vi "Single Ch PI Connect Sequence.vi"(8 "error in (no error)":errorcluster) -> (0 "error out":errorcluster, 2 "PreLaunchStagePos":T1={"Position (SET)"={"XaxesSET"=0.0}, "Position (ACT)"={"PosXACT"=0.0087}} caption="output cluster" {"Position (ACT)"."PosXACT" min=0.0 max=220.0 step=0.1 format="%.2f"; "Position (SET)"."XaxesSET" min=0.0 max=220.0 step=0.1 scale=0.0..220.0}, 3 "Boolean":bool)   [LabVIEW 2020]
uses:
  PI Settings.ctl
  PI Settings Global.vi
  Low Level/Communication.llb/Global1.vi
  Low Level/Communication.llb/Available DLL interfaces.ctl
  Low Level/Communication.llb/Available DLLs.ctl
  Single Ch PI Position.ctl
panel:
  out "Conn. Axes":string[](array[string])
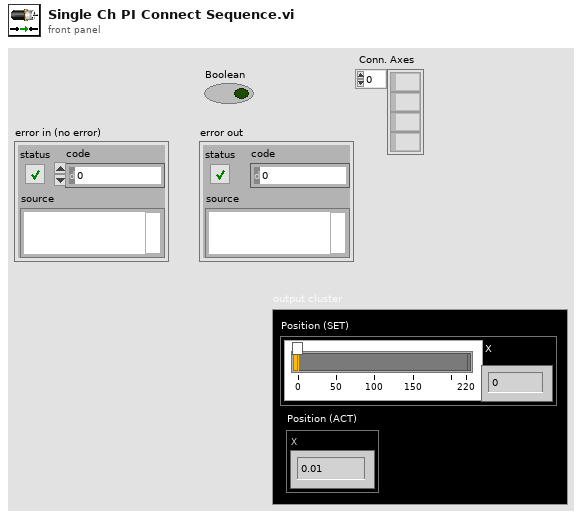
[diagram p1: front panel]
types:
  T1 = typedef "Single Ch PI Position.ctl" = cluster{"Position (SET)":cluster{"XaxesSET":dbl}, "Position (ACT)":cluster{"PosXACT":dbl}}
  T2 = typedef "PI Settings.ctl" = cluster{"System number":i32, "Commanded axes":string[], "Controller error":bool, "Error":errorcluster}
  T3 = typedef "Available DLLs.ctl" = u16
  T4 = typedef "Available DLL interfaces.ctl" = u16
  T5 = cluster{"DLL for Device":T3, "DLL Interface":T4, "Parameter":string}[]
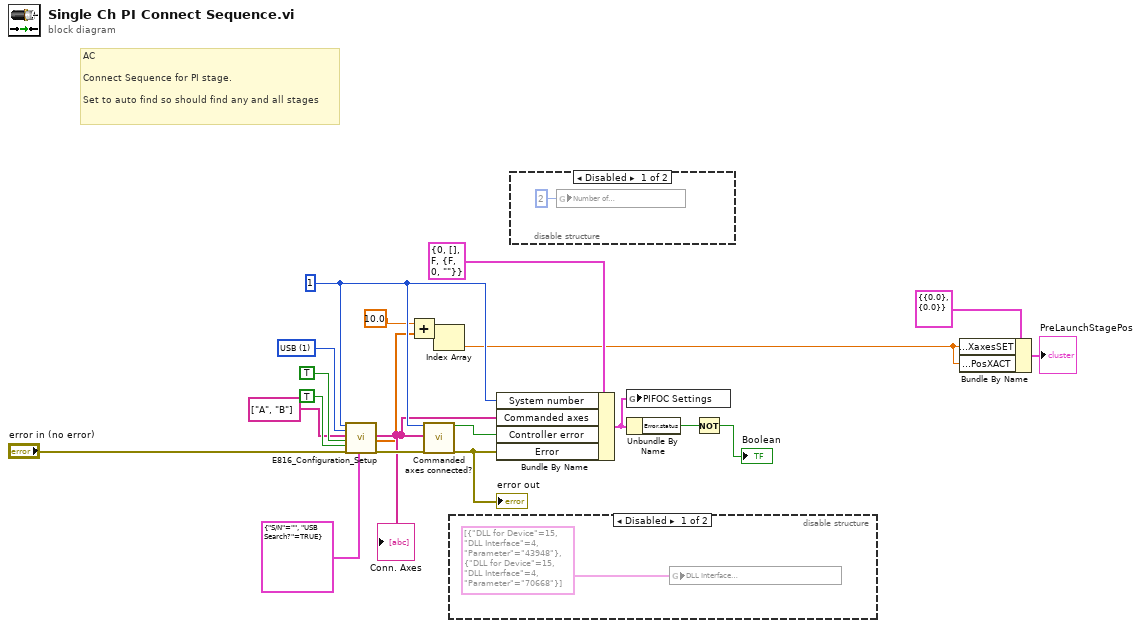
[diagram p0: block diagram]
diagram:
  w13 = u16 1 items=["RS232", "USB"] ("Interface")
  w11 = 1 ("System no.")
  # "AC\n\nConnect Sequence for PI stage.\n\nSet to auto find so should find any and all stages"
  n1 = call "E816_Configuration_Setup.vi"("System no."=w11, "Interface"=w13, "Axes to move"=string[] ["A", "B"], "All axes?"=TRUE, "Change servo \nstatus to ON?"=TRUE ("Use dialog to define\nconnected stages?"), "error in"="error in (no error)", "USB settings"=cluster{"S/N":string, "USB Search?":bool} {"S/N"="", "USB Search?"=TRUE}) -> ("Conn. Axes"=w9:string[], "Position"=w5:dbl[], "error out"=w12:errorcluster)  [unwired: 8 in, 2 out]
  "Conn. Axes" <- w9
  n2 = Add(x=10.0, y=w5) -> (x+y=w2:dbl[])
  n3 = call "Commanded axes connected?.vi"("System no."=w11, "Commanded axes"=w9, "error in"=w12) -> ("Controller error"=w10:bool, "error out"=w18:errorcluster)  [unwired: 15 in]
  "error out" <- w18
  n4 = Index Array(array=w2) -> (element=w3:dbl)  [unwired: 1 in]
  n5 = disable-structure shown="Disabled" {
    frame Disabled {
      n6 = global write "Global1.vi" "DLL Interface\nConfiguration"(T5 [{"DLL for Device"=15, "DLL Interface"=4, "Parameter"="43948"}, {"DLL for Device"=15, "DLL Interface"=4, "Parameter"="70668"}] ("DLL Interface\nConfiguration")) -> ()
    }
    frame Enabled {
    }
  }
  n7 = Bundle By Name(cluster=T2 {"System number"=0, "Commanded axes"=[], "Controller error"=FALSE, "Error"={"status"=FALSE, "code"=0, "source"=""}} ("PIFOC Position 2"), "System number"=w11, "Commanded axes"=w9, "Controller error"=w10, "Error"=w18) -> (w21:T2)
  n8 = disable-structure shown="Disabled" {
    frame Disabled {
      n9 = global write "Global1.vi" "Number of\nsystems"(2 ("Number of\nsystems")) -> ()
    }
    frame Enabled {
    }
  }
  n10 = global write "PI Settings Global.vi" "PIFOC Settings"(w21) -> ()
  n11 = Unbundle By Name(w21) -> ("Error.status"=w15:bool)
  n12 = Not(x=w15) -> (.not. x?=→"Boolean":bool)
  n13 = Bundle By Name(cluster=T1 {"Position (SET)"={"XaxesSET"=0.0}, "Position (ACT)"={"PosXACT"=0.0}} ("Stage Position"), "Position (SET).XaxesSET"=w3, "Position (ACT).PosXACT"=w3) -> (→"PreLaunchStagePos":T1)
